vi "GetDependencies.vi"(8 "error in (no error)":errorcluster, 11 "SMO in":refnum<class "SMO.lvclass">) -> (0 "error out":errorcluster, 2 "Dependencies":refnum<class "Attribute.Dependencies.lvclass">, 3 "SMO out":refnum<class "SMO.lvclass">)   [LabVIEW 2021, in "smo.lvlib" / "SMO.lvclass"]
uses:
  SMO.lvclass
  Support/Attribute.Dependencies/Attribute.Dependencies.lvclass
  SMO.lvclass/SMO.ctl
  ReftoDVR--SMO.vi
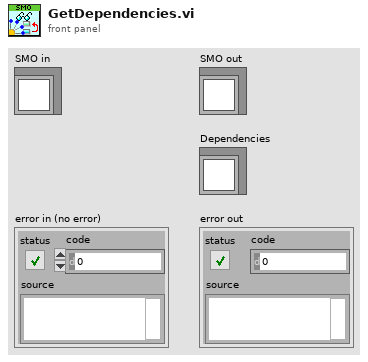
[diagram p1: front panel]
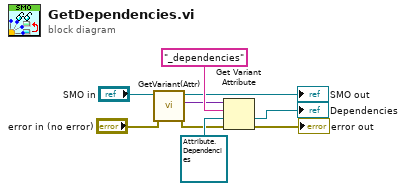
[diagram p0: block diagram]
diagram:
  n1 = call "GetVariant(Attr).vi"("error in (no error)"="error in (no error)", "SMO in"="SMO in") -> ("error out"=w2:errorcluster, "[Attributes]"=w1:variant, "SMO out"=→"SMO out":refnum<class "SMO.lvclass">)  [unwired: 7 in]
  n2 = Get Variant Attribute(Variant=w1, name="_dependencies", default value (empty Variant)=refnum<class "Attribute.Dependencies.lvclass"> refnum ("Attribute.Dependencies.lvclass"), error in=w2) -> (value=→"Dependencies":refnum<class "Attribute.Dependencies.lvclass">, error out=→"error out":errorcluster)  [unwired: 2 out]
